vi "PH_SRDG645.ProcCases.vi"(0 "i ref in":refnum<vi>, 1 "selector":string, 2 "Data":T4, 3 "call cluster":T5={"Object"="", "Selector"="", "CallType"=enum."synchronous", "Async Object"="", "Async Selector"="", "Data Descriptor"="", "Data"=[], "Error #"=0, "Expire"=0}, 5 "error in":errorcluster) -> (14 "i ref out":refnum<vi>, 17 "answer cluster":T5={"Object"="", "Selector"="", "CallType"=enum."synchronous", "Async Object"="", "Async Selector"="", "Data Descriptor"="", "Data"=[], "Error #"=0, "Expire"=0}, 19 "error out":errorcluster)   [LabVIEW 2014, in "PH_SRDG645.lvlib"]
doc: "This method is called by a process from within the default case in the event loop. The methods of a class that are linked to events will be called from THIS method. Add your code here."
uses:
  PH_SRDG645.lvlib
  CS_Core/CSSystem/CoreDefs/CoreDefs.call_type.ctl
  CS_Core/BaseProcess/BaseProcess.descriptor string definition.ctl
  CS_Core/CSSystem/CoreDefs/CoreDefs.rawDataType.ctl
  PH_SRDG645.Trigger.ctl
  PH_SRDG645.Channel Settings.ctl
  CS_Core/CSSystem/CoreLib/CoreLib.byte array 2 int.vi
  CS_Core/CSSystem/CoreLib/CoreLib.byte array 2 double.vi
  CS_Core/CSSystem/CoreLib/CoreLib.string 2 byte array.vi
  CS_Core/CSSystem/CoreLib/CoreLib.byte array 2 short.vi
  CS_Core/CSSystem/CoreLib/CoreLib.lvlib
  CS_Core/BaseProcess/BaseProcess.lvlib
  CS_Core/CAEObj/CAEObj.lvlib
  PH_Basics/PH_PSDBWriter/PH_PSDBWriter.lvlib
  PH_Basics/PH_StatusHandler/PH_StatusHandler.lvlib
panel:
  in  "Output Settings":T1={"Level Offset [V]"=0.0, "Amplitue [V]"=1000.0, "Polarity"=0} {"Polarity" items=["negative", "positive"]}
  in  "Channel Settings":T2={"Delay [s]"=0.0, "relative to"=1000} {"relative to" items=["T0", "T1", "A", "B", "C", "D", "E", "F", "G", "H"]; "Delay [s]" format="%#_12p"}
  in  "Trigger Settings":T3={"Source"=0, "Rate [Hz]"=1000.0, "Level [V]"=1.0} {"Rate [Hz]" format="%#_9p"; "Source" items=["Internal", "External rising edge", "External falling edge", "Single shot external rising edges", "Single shot external falling edges", "Single shot", "Line"]}
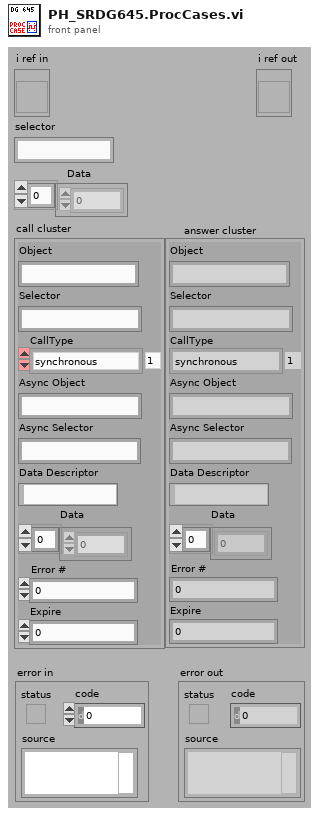
[diagram p1: front panel]
types:
  T1 = cluster{"Level Offset [V]":dbl, "Amplitue [V]":dbl, "Polarity":i32}
  T2 = typedef "PH_SRDG645.lvlib/PH_SRDG645.Channel Settings.ctl" = cluster{"Delay [s]":dbl, "relative to":i32}
  T3 = typedef "PH_SRDG645.lvlib/PH_SRDG645.Trigger.ctl" = cluster{"Source":i32, "Rate [Hz]":dbl, "Level [V]":dbl}
  T4 = typedef "CoreDefs.rawDataType.ctl" = i8[]
  T5 = typedef "CoreDefs.call_type.ctl" = cluster{"Object":string, "Selector":string, "CallType":enum16{"simple", "synchronous", "asynchronous"}, "Async Object":string, "Async Selector":string, "Data Descriptor":T6, "Data":T4, "Error #":i32, "Expire":u32}
  T6 = typedef "BaseProcess.lvlib/BaseProcess.descriptor string definition.ctl" = string
  T7 = typedef "PH_SRDG645.lvlib/PH_SRDG645.i attribute.ctl" = cluster{"GUI Refs":cluster{"Delete":refnum<vi>, "Device Errors":refnum<vi>, "Trigger":refnum<vi>, "Default Name":refnum<vi>, "Firmware Revision":refnum<vi>, "Serial Number":refnum<vi>, "Model":refnum<vi>, "Visa resource name":refnum<vi>}, "Service ID Rate":i32, "Service IDs Channelinfo":i32[], "VISA resource name":refnum<visa-resource-name>, "Device Errors":cluster{"code":i32, "Text":string}[], "Trigger":T3, "Channels":cluster{"T1":T2, "A":T2, "B":T2, "C":T2, "D":T2, "E":T2, "F":T2, "G":T2, "H":T2}, "GUI Refs Channels":refnum<vi>[], "Outputs":cluster{"AB":cluster{"Level Offset [V]":dbl, "Amplitue [V]":dbl, "Polarity":i32}, "CD":cluster{"Level Offset [V]":dbl, "Amplitue [V]":dbl, "Polarity":i32}, "EF":cluster{"Level Offset [V]":dbl, "Amplitue [V]":dbl, "Polarity":i32}, "GH":cluster{"Level Offset [V]":dbl, "Amplitue [V]":dbl, "Polarity":i32}, "T0":cluster{"Level Offset [V]":dbl, "Amplitue [V]":dbl, "Polarity":i32}}, "GUI Refs Outputs":refnum<vi>[], "Serial Number":string, "Firmweare Revision":string, "Model":string}
  T8 = typedef "PH_PSDBWriter.lvlib/PH_PSDBWriter.PHELIX-Subsystems.ctl" = i32
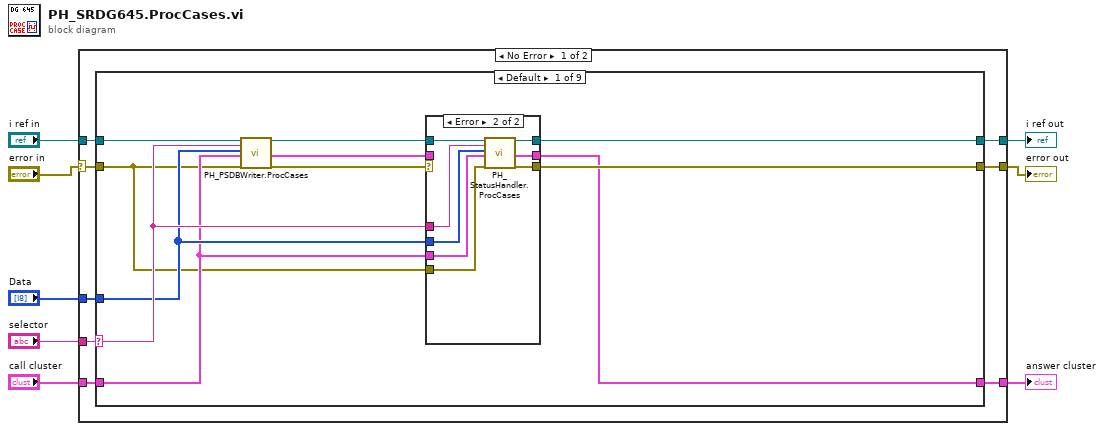
[diagram p0: block diagram]
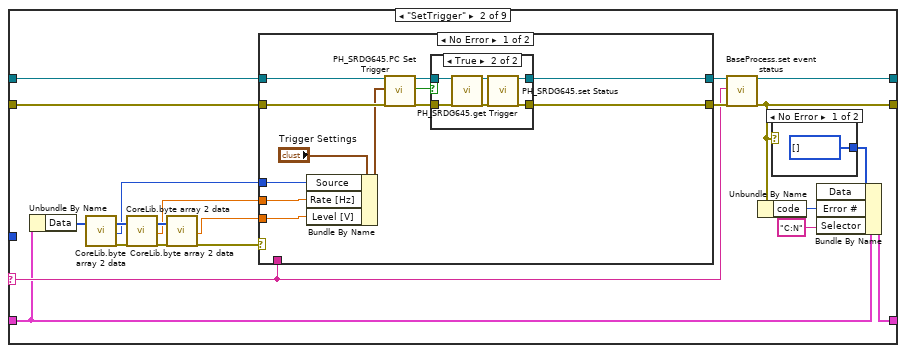
[diagram p3: hidden frame]
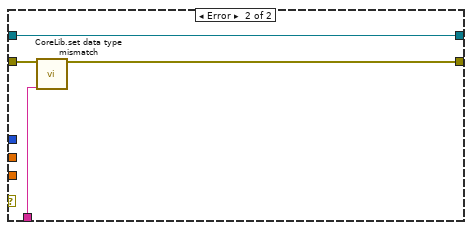
[diagram p5: hidden frame]
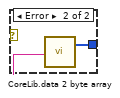
[diagram p6: hidden frame]
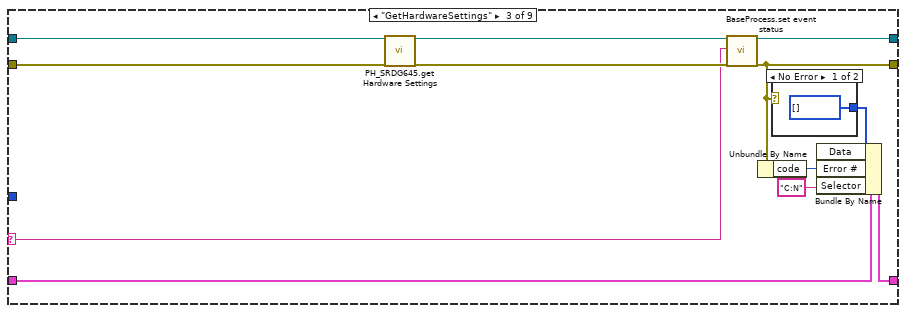
[diagram p7: hidden frame]
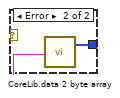
[diagram p8: hidden frame]
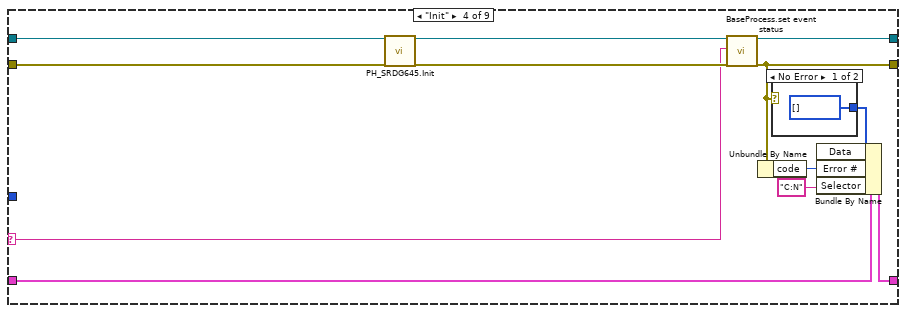
[diagram p9: hidden frame]
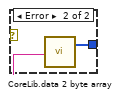
[diagram p10: hidden frame]
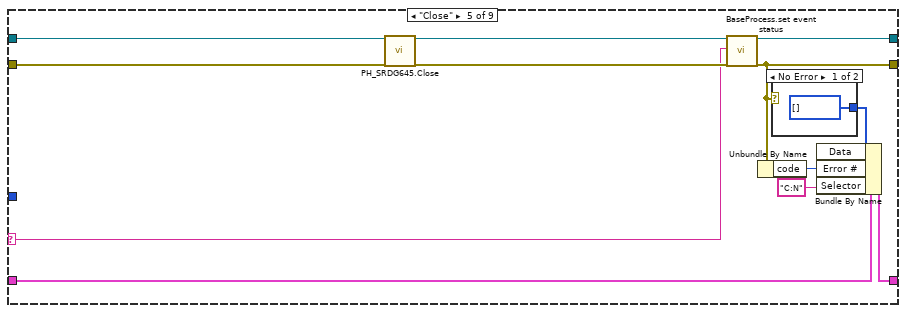
[diagram p11: hidden frame]
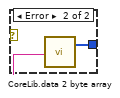
[diagram p12: hidden frame]
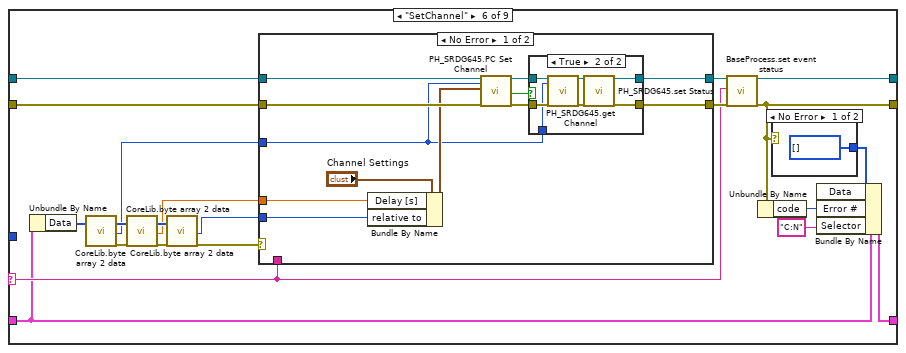
[diagram p13: hidden frame]
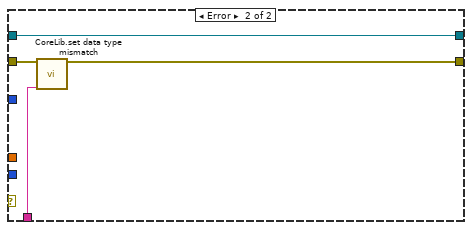
[diagram p15: hidden frame]
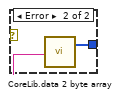
[diagram p16: hidden frame]
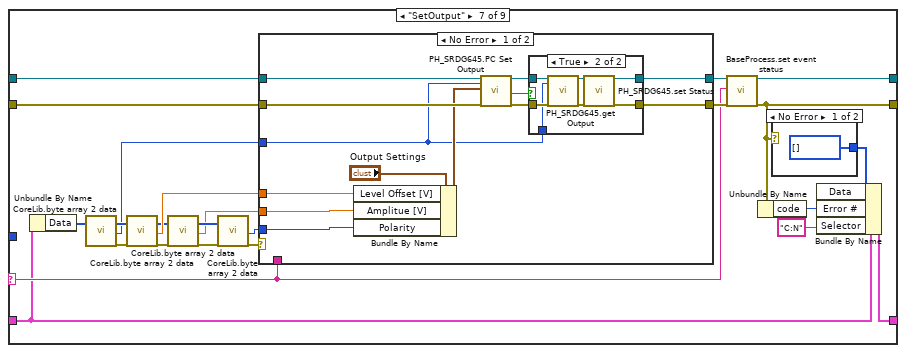
[diagram p17: hidden frame]
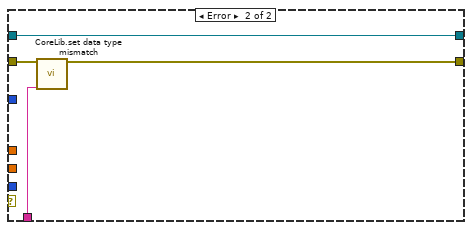
[diagram p19: hidden frame]
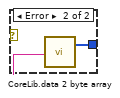
[diagram p20: hidden frame]
diagram:
  n1 = case shown="No Error" "error in" {
    selector: "error in" -> [w9 w325]
    tunnel: "selector" -> [w16 _]
    tunnel: [w15 w326] -> w7
    tunnel: "call cluster" -> [w14 w326]
    tunnel: "i ref in" -> [w13 w327]
    tunnel: [w12 w327] -> w4
    tunnel: [w11 w325] -> w3
    tunnel: "Data" -> [w10 _]
    frame No Error {
      n2 = case shown="Default" w16 {
        selector: w16 -> [w20 w46 w91 w107 w123 w143 w198 w240 w282]
        tunnel: w13 -> [w27 w49 w94 w110 w126 w146 w201 w244 w284]
        tunnel: [w25 w48 w93 w109 w125 w145 w200 w252 w295] -> w12
        tunnel: w14 -> [w18 w44 w89 w105 w121 w141 w196 w241 w292]
        tunnel: [w23 w43 w88 w104 w120 w140 w195 w250 w293] -> w15
        tunnel: w9 -> [w17 w47 w92 w108 w124 w144 w199 w245 w283]
        tunnel: [w24 w45 w90 w106 w122 w142 w197 w251 w294] -> w11
        tunnel: w10 -> [w19 _ _ _ _ _ _ _ w281]
        frame Default {
          # "In the default case, always call the ProcCase method of the parent class"
          n3 = call "PH_PSDBWriter.ProcCases.vi"("i ref in"=w27, "selector"=w20, "Data"=w19, "call cluster"=w18, "error in"=w17) -> ("i ref out"=w26:refnum<vi>, "answer cluster"=w21:T5, "error out"=w22:errorcluster)  [unwired: 12 in]
          n4 = case shown="Error" w22 {
            selector: w22 -> [w29 _]
            tunnel: [w29 w38] -> w24
            tunnel: w26 -> [w30 w37]
            tunnel: [w30 w36] -> w25
            tunnel: [w28 w35] -> w23
            tunnel: w17 -> [_ w34]
            tunnel: w18 -> [_ w33]
            tunnel: w19 -> [_ w32]
            tunnel: w20 -> [_ w31]
            tunnel: w21 -> [w28 _]
            frame No Error {
            }
            frame Error {
              n5 = call "PH_StatusHandler.ProcCases.vi"("i ref in"=w37, "selector"=w31, "Data"=w32, "call cluster"=w33, "error in (no error)"=w34) -> ("i ref out"=w36:refnum<vi>, "answer cluster"=w35:T5, "error out"=w38:errorcluster)  [unwired: 12 in]
            }
          }
        }
        frame "SetTrigger" {
          n6 = Unbundle By Name(w44) -> ("Data"=w50:T4)
          n7 = call-poly "CoreLib.byte array 2 data.vi"("byteArray"=w50) -> ("byteArray out"=w52:T4, "i32"=w42:i32, "error out"=w54:errorcluster)  [unwired: 16 in]
          n8 = call-poly "CoreLib.byte array 2 data.vi"("byteArray"=w52, "error in (no error)"=w54) -> ("byteArray out"=w51:T4, "d64"=w41:dbl, "error out"=w53:errorcluster)  [unwired: 15 in]
          n9 = call-poly "CoreLib.byte array 2 data.vi"("byteArray"=w51, "error in (no error)"=w53) -> ("d64"=w40:dbl, "error out"=w39:errorcluster)  [unwired: 15 in, 1 out]
          n10 = case shown="No Error" w39 {
            tunnel: [w68 w83] -> w55
            tunnel: w49 -> [w71 w83]
            tunnel: w47 -> [w70 w82]
            tunnel: [w67 w81] -> w56
            tunnel: w46 -> [_ w80]
            tunnel: w42 -> [w62 _]
            tunnel: w41 -> [w63 _]
            tunnel: w40 -> [w64 _]
            frame No Error {
              n11 = Bundle By Name(cluster="Trigger Settings", "Source"=w62, "Rate [Hz]"=w63, "Level [V]"=w64) -> (w65:T3)
              n12 = call "PH_SRDG645.PC Set Trigger.vi"("i ref in"=w71, "Trigger Settings"=w65, "error IO"=w70) -> ("i ref out"=w61:refnum<vi>, "something changed?"=w60:bool, "error out"=w69:errorcluster)  [unwired: 14 in]
              n13 = case shown="True" w60 {
                tunnel: w69 -> [w72 w79]
                tunnel: [w73 w78] -> w68
                tunnel: [w72 w77] -> w67
                tunnel: w61 -> [w73 w75]
                frame False {
                }
                frame True {
                  n14 = call "PH_SRDG645.get Trigger.vi"("i ref in"=w75, "error IO"=w79) -> ("i ref out"=w74:refnum<vi>, "error out"=w76:errorcluster)  [unwired: 16 in]
                  n15 = call "PH_SRDG645.set Status.vi"("i ref in"=w74, "error in"=w76) -> ("i ref out"=w78:refnum<vi>, "error out"=w77:errorcluster)  [unwired: 16 in]
                }
              }
            }
            frame Error {
              n16 = call "CoreLib.set data type mismatch.vi"("error in (no error)"=w82, "error source"=w80) -> ("error out"=w81:errorcluster)  [unwired: 17 in]
            }
          }
          n17 = call "BaseProcess.set event status.vi"("i ref in"=w55, "EventStatus"=w46, "error in (no error)"=w56) -> ("i ref out"=w48:refnum<vi>, "error out"=w45:errorcluster)  [unwired: 14 in, 1 out]
          n18 = Unbundle By Name(w45) -> ("code"=w59:i32)
          n19 = case shown="No Error" w45 {
            selector: w45 -> [_ w87]
            tunnel: [T4 [] ("byteArray out") w85] -> w58
            frame No Error {
            }
            frame Error {
              n20 = Unbundle By Name(w87) -> ("source"=w86:string)
              n21 = call-poly "CoreLib.data 2 byte array.vi"("string"=w86) -> ("byteArray out"=w85:T4)  [unwired: 18 in]
            }
          }
          n22 = Bundle By Name(cluster=w44, "Data"=w58, "Error #"=w59, "Selector"="C:N") -> (w43:T5)
        }
        frame "GetHardwareSettings" {
          n23 = call "PH_SRDG645.get Hardware Settings.vi"("i ref in"=w94, "error in"=w92) -> ("i ref out"=w95:refnum<vi>, "error out"=w96:errorcluster)  [unwired: 16 in]
          n24 = call "BaseProcess.set event status.vi"("i ref in"=w95, "EventStatus"=w91, "error in (no error)"=w96) -> ("i ref out"=w93:refnum<vi>, "error out"=w90:errorcluster)  [unwired: 14 in, 1 out]
          n25 = Unbundle By Name(w90) -> ("code"=w99:i32)
          n26 = case shown="No Error" w90 {
            selector: w90 -> [_ w103]
            tunnel: [T4 [] ("byteArray out") w101] -> w98
            frame No Error {
            }
            frame Error {
              n27 = Unbundle By Name(w103) -> ("source"=w102:string)
              n28 = call-poly "CoreLib.data 2 byte array.vi"("string"=w102) -> ("byteArray out"=w101:T4)  [unwired: 18 in]
            }
          }
          n29 = Bundle By Name(cluster=w89, "Data"=w98, "Error #"=w99, "Selector"="C:N") -> (w88:T5)
        }
        frame "Init" {
          n30 = call "PH_SRDG645.Init.vi"("i ref in"=w110, "error in"=w108) -> ("i ref out"=w111:refnum<vi>, "error out"=w112:errorcluster)  [unwired: 16 in]
          n31 = call "BaseProcess.set event status.vi"("i ref in"=w111, "EventStatus"=w107, "error in (no error)"=w112) -> ("i ref out"=w109:refnum<vi>, "error out"=w106:errorcluster)  [unwired: 14 in, 1 out]
          n32 = Unbundle By Name(w106) -> ("code"=w115:i32)
          n33 = case shown="No Error" w106 {
            selector: w106 -> [_ w119]
            tunnel: [T4 [] ("byteArray out") w117] -> w114
            frame No Error {
            }
            frame Error {
              n34 = Unbundle By Name(w119) -> ("source"=w118:string)
              n35 = call-poly "CoreLib.data 2 byte array.vi"("string"=w118) -> ("byteArray out"=w117:T4)  [unwired: 18 in]
            }
          }
          n36 = Bundle By Name(cluster=w105, "Data"=w114, "Error #"=w115, "Selector"="C:N") -> (w104:T5)
        }
        frame "Close" {
          n37 = call "PH_SRDG645.Close.vi"("i ref in"=w126, "error in"=w124) -> ("i ref out"=w127:refnum<vi>, "error out"=w128:errorcluster)  [unwired: 16 in]
          n38 = call "BaseProcess.set event status.vi"("i ref in"=w127, "EventStatus"=w123, "error in (no error)"=w128) -> ("i ref out"=w125:refnum<vi>, "error out"=w122:errorcluster)  [unwired: 14 in, 1 out]
          n39 = Unbundle By Name(w122) -> ("code"=w131:i32)
          n40 = case shown="No Error" w122 {
            selector: w122 -> [_ w135]
            tunnel: [T4 [] ("byteArray out") w133] -> w130
            frame No Error {
            }
            frame Error {
              n41 = Unbundle By Name(w135) -> ("source"=w134:string)
              n42 = call-poly "CoreLib.data 2 byte array.vi"("string"=w134) -> ("byteArray out"=w133:T4)  [unwired: 18 in]
            }
          }
          n43 = Bundle By Name(cluster=w121, "Data"=w130, "Error #"=w131, "Selector"="C:N") -> (w120:T5)
        }
        frame "SetChannel" {
          n44 = Unbundle By Name(w141) -> ("Data"=w147:T4)
          n45 = call-poly "CoreLib.byte array 2 data.vi"("byteArray"=w147) -> ("byteArray out"=w149:T4, "i32"=w139:i32, "error out"=w151:errorcluster)  [unwired: 16 in]
          n46 = call-poly "CoreLib.byte array 2 data.vi"("byteArray"=w149, "error in (no error)"=w151) -> ("byteArray out"=w148:T4, "d64"=w138:dbl, "error out"=w150:errorcluster)  [unwired: 15 in]
          n47 = call-poly "CoreLib.byte array 2 data.vi"("byteArray"=w148, "error in (no error)"=w150) -> ("i32"=w137:i32, "error out"=w136:errorcluster)  [unwired: 15 in, 1 out]
          n48 = case shown="No Error" w136 {
            tunnel: [w165 w181] -> w152
            tunnel: w146 -> [w168 w181]
            tunnel: w144 -> [w167 w180]
            tunnel: [w164 w179] -> w153
            tunnel: w143 -> [_ w178]
            tunnel: w139 -> [w157 _]
            tunnel: w138 -> [w160 _]
            tunnel: w137 -> [w161 _]
            frame No Error {
              n49 = Bundle By Name(cluster="Channel Settings", "Delay [s]"=w160, "relative to"=w161) -> (w162:T2)
              n50 = call "PH_SRDG645.PC Set Channel.vi"("i ref in"=w168, "Channel to set"=w157, "Channel Settings"=w162, "error IO"=w167) -> ("i ref out"=w159:refnum<vi>, "Something changed?"=w158:bool, "error out"=w166:errorcluster)  [unwired: 13 in]
              n51 = case shown="True" w158 {
                tunnel: w166 -> [w169 w177]
                tunnel: [w170 w176] -> w165
                tunnel: [w169 w175] -> w164
                tunnel: w159 -> [w170 w173]
                tunnel: w157 -> [_ w171]
                frame False {
                }
                frame True {
                  n52 = call "PH_SRDG645.get Channel.vi"("i ref in"=w173, "Channel (T0)"=w171, "error IO"=w177) -> ("i ref out"=w172:refnum<vi>, "error out"=w174:errorcluster)  [unwired: 15 in]
                  n53 = call "PH_SRDG645.set Status.vi"("i ref in"=w172, "error in"=w174) -> ("i ref out"=w176:refnum<vi>, "error out"=w175:errorcluster)  [unwired: 16 in]
                }
              }
            }
            frame Error {
              n54 = call "CoreLib.set data type mismatch.vi"("error in (no error)"=w180, "error source"=w178) -> ("error out"=w179:errorcluster)  [unwired: 17 in]
            }
          }
          n55 = call "BaseProcess.set event status.vi"("i ref in"=w152, "EventStatus"=w143, "error in (no error)"=w153) -> ("i ref out"=w145:refnum<vi>, "error out"=w142:errorcluster)  [unwired: 14 in, 1 out]
          n56 = Unbundle By Name(w142) -> ("code"=w156:i32)
          n57 = case shown="No Error" w142 {
            selector: w142 -> [_ w185]
            tunnel: [T4 [] ("byteArray out") w183] -> w155
            frame No Error {
            }
            frame Error {
              n58 = Unbundle By Name(w185) -> ("source"=w184:string)
              n59 = call-poly "CoreLib.data 2 byte array.vi"("string"=w184) -> ("byteArray out"=w183:T4)  [unwired: 18 in]
            }
          }
          n60 = Bundle By Name(cluster=w141, "Data"=w155, "Error #"=w156, "Selector"="C:N") -> (w140:T5)
        }
        frame "SetOutput" {
          n61 = Unbundle By Name(w196) -> ("Data"=w202:T4)
          n62 = call-poly "CoreLib.byte array 2 data.vi"("byteArray"=w202) -> ("byteArray out"=w203:T4, "i32"=w194:i32, "error out"=w204:errorcluster)  [unwired: 16 in]
          n63 = call-poly "CoreLib.byte array 2 data.vi"("byteArray"=w203, "error in (no error)"=w204) -> ("byteArray out"=w188:T4, "d64"=w193:dbl, "error out"=w190:errorcluster)  [unwired: 15 in]
          n64 = call-poly "CoreLib.byte array 2 data.vi"("byteArray"=w188, "error in (no error)"=w190) -> ("byteArray out"=w187:T4, "d64"=w186:dbl, "error out"=w189:errorcluster)  [unwired: 15 in]
          n65 = call-poly "CoreLib.byte array 2 data.vi"("byteArray"=w187, "error in (no error)"=w189) -> ("i32"=w192:i32, "error out"=w191:errorcluster)  [unwired: 15 in, 1 out]
          n66 = case shown="No Error" w191 {
            tunnel: [w219 w235] -> w205
            tunnel: w201 -> [w222 w235]
            tunnel: w199 -> [w221 w234]
            tunnel: [w218 w233] -> w206
            tunnel: w198 -> [_ w232]
            tunnel: w194 -> [w212 _]
            tunnel: w193 -> [w215 _]
            tunnel: w192 -> [w211 _]
            tunnel: w186 -> [w210 _]
            frame No Error {
              n67 = Bundle By Name(cluster="Output Settings", "Level Offset [V]"=w215, "Amplitue [V]"=w210, "Polarity"=w211) -> (w216:T1)
              n68 = call "PH_SRDG645.PC Set Output.vi"("i ref in"=w222, "Output to set"=w212, "Output Settings"=w216, "error IO"=w221) -> ("i ref out"=w214:refnum<vi>, "Something changed?"=w213:bool, "error out"=w220:errorcluster)  [unwired: 13 in]
              n69 = case shown="True" w213 {
                tunnel: w220 -> [w223 w231]
                tunnel: [w224 w230] -> w219
                tunnel: [w223 w229] -> w218
                tunnel: w214 -> [w224 w227]
                tunnel: w212 -> [_ w225]
                frame False {
                }
                frame True {
                  n70 = call "PH_SRDG645.get Output.vi"("i ref in"=w227, "Output BNC (T0)"=w225, "error IO"=w231) -> ("i ref out"=w226:refnum<vi>, "error out"=w228:errorcluster)  [unwired: 15 in]
                  n71 = call "PH_SRDG645.set Status.vi"("i ref in"=w226, "error in"=w228) -> ("i ref out"=w230:refnum<vi>, "error out"=w229:errorcluster)  [unwired: 16 in]
                }
              }
            }
            frame Error {
              n72 = call "CoreLib.set data type mismatch.vi"("error in (no error)"=w234, "error source"=w232) -> ("error out"=w233:errorcluster)  [unwired: 17 in]
            }
          }
          n73 = call "BaseProcess.set event status.vi"("i ref in"=w205, "EventStatus"=w198, "error in (no error)"=w206) -> ("i ref out"=w200:refnum<vi>, "error out"=w197:errorcluster)  [unwired: 14 in, 1 out]
          n74 = Unbundle By Name(w197) -> ("code"=w209:i32)
          n75 = case shown="No Error" w197 {
            selector: w197 -> [_ w239]
            tunnel: [T4 [] ("byteArray out") w237] -> w208
            frame No Error {
            }
            frame Error {
              n76 = Unbundle By Name(w239) -> ("source"=w238:string)
              n77 = call-poly "CoreLib.data 2 byte array.vi"("string"=w238) -> ("byteArray out"=w237:T4)  [unwired: 18 in]
            }
          }
          n78 = Bundle By Name(cluster=w196, "Data"=w208, "Error #"=w209, "Selector"="C:N") -> (w195:T5)
        }
        frame "Control Remote" {
          n79 = Unbundle By Name(w241) -> ("Data"=w246:T4)
          n80 = call-poly "CoreLib.byte array 2 data.vi"("byteArray"=w246) -> ("i16"=w247:i16, "error out"=w249:errorcluster)  [unwired: 16 in, 1 out]
          n81 = Greater Than 0?(x=w247) -> (x > 0?=w248:bool)
          n82 = case shown="No Error" w249 {
            tunnel: [w258 w276] -> w243
            tunnel: w244 -> [w264 w276]
            tunnel: w245 -> [w263 w275]
            tunnel: [w259 w274] -> w242
            tunnel: w240 -> [_ w273]
            tunnel: w248 -> [w260 _]
            frame No Error {
              n83 = call "PH_SRDG645.get i attribute.vi"("i ref in"=w264, "error in (no error)"=w263) -> ("i ref out"=w258:refnum<vi>, "i attribute"=w262:T7, "error out"=w261:errorcluster)  [unwired: 15 in]
              n84 = Unbundle By Name(w262) -> ("GUI Refs.Delete"=w257:refnum<vi>)
              n85 = Not A Number/Path/Refnum?(number/path/refnum=w257) -> (NaN/Path/Refnum?=w256:bool)
              n86 = case shown="False" w256 {
                tunnel: w257 -> [w269 _]
                tunnel: w261 -> [w268 w272]
                tunnel: [w267 w272] -> w259
                tunnel: w260 -> [w266 _]
                frame False {
                  n87 = case shown="True" w266 {
                    tunnel: [0 2] -> w265
                    frame False {
                    }
                    frame True {
                    }
                  }
                  n88 = property class="Bool"(reference=w269, error in=w268, "Disabled"=w265) -> (error out=w267:errorcluster)  [unwired: 1 out]
                }
                frame True {
                }
              }
            }
            frame Error {
              n89 = call "CoreLib.set data type mismatch.vi"("error in (no error)"=w275, "error source"=w273) -> ("error out"=w274:errorcluster)  [unwired: 17 in]
            }
          }
          n90 = call "BaseProcess.set event status.vi"("i ref in"=w243, "EventStatus"=w240, "error in (no error)"=w242) -> ("i ref out"=w252:refnum<vi>, "error out"=w251:errorcluster)  [unwired: 14 in, 1 out]
          n91 = Unbundle By Name(w251) -> ("code"=w255:i32)
          n92 = case shown="No Error" w251 {
            selector: w251 -> [_ w280]
            tunnel: [T4 [] ("byteArray out") w278] -> w254
            frame No Error {
            }
            frame Error {
              n93 = Unbundle By Name(w280) -> ("source"=w279:string)
              n94 = call-poly "CoreLib.data 2 byte array.vi"("string"=w279) -> ("byteArray out"=w278:T4)  [unwired: 18 in]
            }
          }
          n95 = Bundle By Name(cluster=w241, "Data"=w254, "Error #"=w255, "Selector"="C:N") -> (w250:T5)
        }
        frame "_set_PSDB_Data" {
          n96 = call "CAEObj.unfold trend data.vi"("i ref in"=w284, "raw trend data"=w281) -> ("quality"=w287:i32, "no link"=w290:bool, "data"=w288:i8[], "typeDescriptor"=w289:string, "error out"=w291:errorcluster)  [unwired: 9 in, 4 out]
          n97 = case shown="No Error" w291 {
            tunnel: w283 -> [w310 w320]
            tunnel: [w309 w319] -> w286
            tunnel: [w308 w320] -> w285
            tunnel: w284 -> [w306 w319]
            tunnel: w290 -> [w300 _]
            tunnel: w289 -> [w301 _]
            tunnel: w288 -> [w302 _]
            tunnel: w287 -> [w303 _]
            frame No Error {
              n98 = call "PH_PSDBWriter.get Subsystem DIM Service.vi"("no link"=w300, "typeDescriptor"=w301, "data"=w302, "quality"=w303) -> ("PHELIX Subsystems"=w299:T8)
              n99 = call "PH_PSDBWriter.check PSDB writing condition.vi"("i ref in"=w306, "wanted Subsystem"=w299, "error IO"=w310) -> ("i ref out"=w305:refnum<vi>, "write PSDB?"=w304:bool, "error out"=w307:errorcluster)  [unwired: 14 in]
              n100 = case shown="True" w304 {
                tunnel: w307 -> [w311 w318]
                tunnel: [w312 w315] -> w309
                tunnel: [w311 w313] -> w308
                tunnel: w305 -> [w312 w317]
                frame False {
                }
                frame True {
                  n101 = call "PH_SRDG645.PC Write PSDB.vi"("i ref in"=w317, "error IO"=w318) -> ("i ref out"=w316:refnum<vi>, "error out"=w314:errorcluster)  [unwired: 16 in]
                  n102 = call "PH_PSDBWriter.evt call write PSDB.vi"("i ref in"=w316, "error in (no error)"=w314) -> ("i ref out"=w315:refnum<vi>, "error out"=w313:errorcluster)  [unwired: 16 in]
                }
              }
            }
            frame Error {
            }
          }
          n103 = call "BaseProcess.set event status.vi"("i ref in"=w286, "EventStatus"=w282, "error in (no error)"=w285) -> ("i ref out"=w295:refnum<vi>, "error out"=w294:errorcluster)  [unwired: 14 in, 1 out]
          n104 = Unbundle By Name(w294) -> ("code"=w298:i32)
          n105 = case shown="No Error" w294 {
            selector: w294 -> [_ w324]
            tunnel: [T4 [] ("byteArray out") w322] -> w297
            frame No Error {
            }
            frame Error {
              n106 = Unbundle By Name(w324) -> ("source"=w323:string)
              n107 = call-poly "CoreLib.data 2 byte array.vi"("string"=w323) -> ("byteArray out"=w322:T4)  [unwired: 18 in]
            }
          }
          n108 = Bundle By Name(cluster=w292, "Data"=w297, "Error #"=w298, "Selector"="C:N") -> (w293:T5)
        }
      }
    }
    frame Error {
    }
  }
  "answer cluster" <- w7
  "i ref out" <- w4
  "error out" <- w3
